vi "edittest parse state keys.vi"(8 "error in (no error)":errorcluster, 9 "REFQUERY (empty)":T1, 10 "POST (empty)":T1, 11 "Template Keys In (empty)":T1) -> (0 "error out":errorcluster, 3 "Template Keys Out":T1)   [LabVIEW 2011]
uses:
  Addons/internet/utils/keyedarr.llb/Keyed Array.ctl
  Addons/internet/utils/strutil.llb/Case Matching.ctl
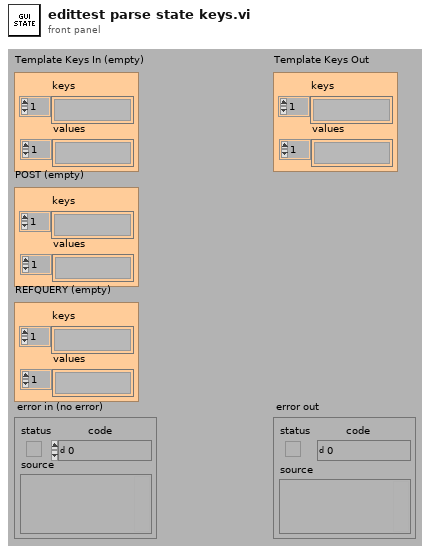
[diagram p1: front panel]
types:
  T1 = typedef "Keyed Array.ctl" = cluster{"keys":string[], "values":string[]}
  T2 = typedef "Case Matching.ctl" = enum16{"a != A", "a == A", "system"}
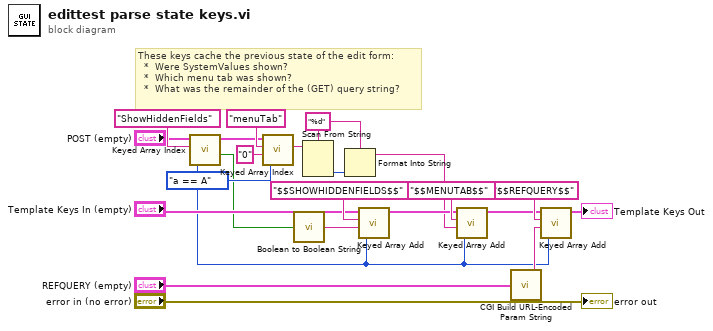
[diagram p0: block diagram]
diagram:
  w4 = "%d" ("format string")
  w3 = Case_Matching."a == A" ("case matching (sensitive)")
  # "These keys cache the previous state of the edit form:\n  *  Were SystemValues shown?\n  *  Which menu tab was shown?\n  *  What was the remainder of the (GET) query string?"
  n1 = call "Keyed Array Index.vi"("case matching (sensitive)"=w3, "key"="ShowHiddenFields", "array in"="POST (empty)") -> ("valid key"=w1:bool, "duplicate array"=w20:T1)  [unwired: 1 in, 2 out]
  n2 = call "Keyed Array Index.vi"("case matching (sensitive)"=w3, "default value"="0", "key"="menuTab", "array in"=w20) -> ("value"=w19:string)  [unwired: 3 out]
  n3 = call "Boolean to Boolean String.vi"("Boolean"=w1) -> ("Boolean string"=w2:string)  [unwired: 1 in]
  n4 = Scan From String(format string=w4, input string=w19) -> (output 1=w18:i32)  [unwired: 2 in, 4 out]
  n5 = Format Into String(format string=w4, w18) -> (resulting string=w13:string)  [unwired: 2 in, 1 out]
  n6 = call "Keyed Array Add.vi"("case matching (sensitive)"=w3, "value"=w2, "key"="$$SHOWHIDDENFIELDS$$", "array in"="Template Keys In (empty)") -> ("array out"=w14:T1)  [unwired: 3 out]
  n7 = call "Keyed Array Add.vi"("case matching (sensitive)"=w3, "value"=w13, "key"="$$MENUTAB$$", "array in"=w14) -> ("array out"=w10:T1)  [unwired: 3 out]
  n8 = call "CGI Build URL-Encoded Param String.vi"("params"="REFQUERY (empty)") -> ("url-encoded param string"=w12:string)
  n9 = call "Keyed Array Add.vi"("case matching (sensitive)"=w3, "value"=w12, "key"="$$REFQUERY$$", "array in"=w10) -> ("array out"=→"Template Keys Out":T1)  [unwired: 3 out]
  "error out" <- "error in (no error)"
